vi "Read n Register Stop uService GUI Event Handler .vi"(8 "error in (no error)":errorcluster, 11 "uService Template in":refnum<class "Father of all uServices.lvclass">) -> (0 "error out":errorcluster, 2 "Stop uService GUI Event Ref":refnum<event-registration>, 3 "uService Template out":refnum<class "Father of all uServices.lvclass">)   [LabVIEW 2026, in "TALOS.lvlib" / "Father of all uServices.lvlib" / "Father of all uServices.lvclass"]
uses:
  Father of all uServices.lvclass
  Father of all uServices.lvclass/Father of all uServices.ctl
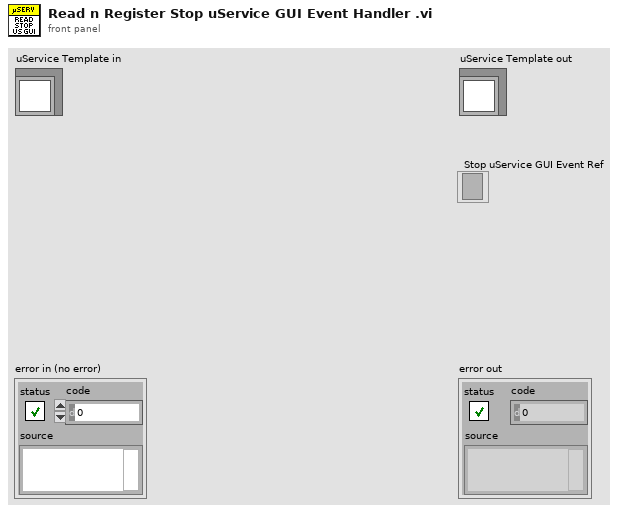
[diagram p1: front panel]
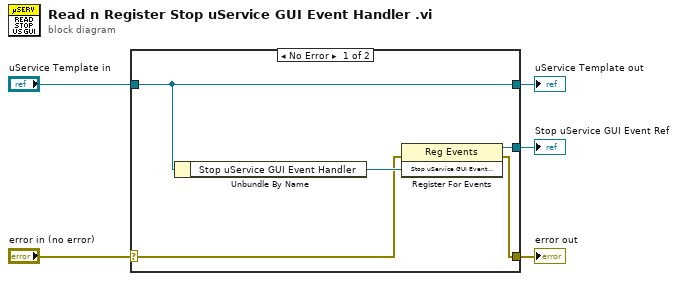
[diagram p0: block diagram]
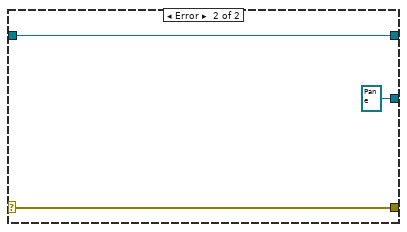
[diagram p2: hidden frame]
diagram:
  n1 = case shown="No Error" "error in (no error)" {
    selector: "error in (no error)" -> [w7 w12]
    tunnel: [w6 w12] -> w4
    tunnel: [w10 w13] -> w2
    tunnel: "uService Template in" -> [w10 w13]
    tunnel: [w8 refnum<event-registration> refnum ("Event Registration Refnum")] -> w1
    frame No Error {
      n2 = Unbundle By Name(w10) -> ("Stop uService GUI Event Handler"=w9:refnum<user-event>)
      n3 = register-events(error in=w7, w9) -> (reference out=w8:refnum<event-registration>, error out=w6:errorcluster)  [unwired: 1 in]
    }
    frame Error {
    }
  }
  "error out" <- w4
  "uService Template out" <- w2
  "Stop uService GUI Event Ref" <- w1
